vi "Add Entry.vi"(5 "Extra Info":T1, 6 "Parent (None)":string[](array[string]), 7 "Name Prefix (none)":string, 8 "error in (no error)":errorcluster, 9 "Columns":string[](array[string]), 10 "Name":string, 11 "Tree Map in":refnum<class "Tree Map.lvclass">) -> (0 "error out":errorcluster, 3 "Tree Map out":refnum<class "Tree Map.lvclass">, 4 "Hierarchy":string[](array[string]))   [LabVIEW 2020, in "Tree Map.lvlib" / "Tree Map.lvclass"]
uses:
  Tree Map.lvclass
  Extra Entry Info.ctl
  Tree Entry.ctl
  Tree Map.lvclass/Tree Map.ctl
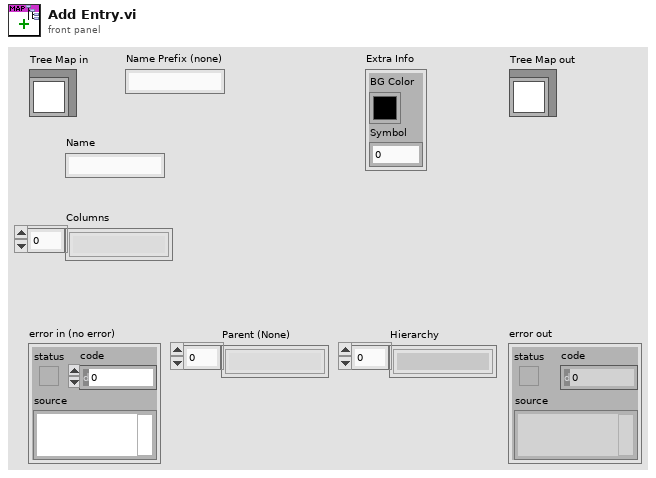
[diagram p1: front panel]
types:
  T1 = typedef "Tree Map.lvlib/Tree Map.lvclass/Extra Entry Info.ctl" = cluster{"BG Color":u32, "Symbol":i32}
  T2 = typedef "Tree Map.lvlib/Tree Map.lvclass/Tree Entry.ctl" = cluster{"Hierarchy":string[], "Name":string, "Columns":string[], "Leaf":bool, "Extra":T1}
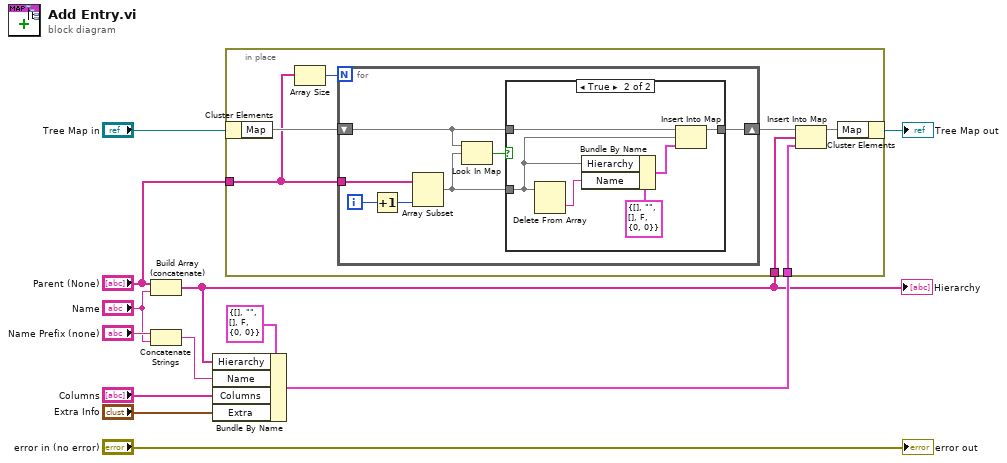
[diagram p0: block diagram]
diagram:
  n1 = Build Array (concatenate)("Parent (None)", "Name") -> (w4:string[])
  "Hierarchy" <- w4
  n2 = Concatenate Strings("Name Prefix (none)", "Name") -> (w8:string)
  n3 = Bundle By Name(cluster=T2 {"Hierarchy"=[], "Name"="", "Columns"=[], "Leaf"=FALSE, "Extra"={"BG Color"=0, "Symbol"=0}} ("Tree Entry"), "Hierarchy"=w4, "Name"=w8, "Columns"="Columns", "Extra"="Extra Info") -> (w5:T2)
  n4 = in-place {
    in-place-border: w5 -> [w19]
    in-place-border: w4 -> [w18]
    in-place-border: "Parent (None)" -> [w14]
    n5 = in-place-cluster #1("Tree Map in") -> ("Map"=w16:map{string[], T2})
    n6 = Array Size(array=w14) -> (size(s)=w13:i32)
    n7 = for {
      N: w13 -> [_]
      shift-right: [w21] -> w15
      shift-left: w16 -> [w23]
      tunnel: w14 -> [w26]
      i -> [w25]
      n8 = Increment(x=w25) -> (x+1=w20:i32)
      n9 = Array Subset(array=w26, length=w20) -> (w22:string[])  [unwired: 1 in]
      n10 = Look In Map(map=w23, key=w22) -> (key not found?=w24:bool)  [unwired: 1 in, 1 out]
      n11 = case shown="True" w24 {
        tunnel: w23 -> [w27 w33]
        tunnel: w22 -> [_ w29]
        tunnel: [w27 w32] -> w21
        frame False {
        }
        frame True {
          n12 = Delete From Array(array=w29) -> (deleted portion=w28:string)  [unwired: 2 in, 1 out]
          n13 = Bundle By Name(cluster=T2 {"Hierarchy"=[], "Name"="", "Columns"=[], "Leaf"=FALSE, "Extra"={"BG Color"=0, "Symbol"=0}} ("value"), "Hierarchy"=w29, "Name"=w28) -> (w30:T2)
          n14 = Insert Into Map(map in=w33, key=w29, value=w30) -> (map out=w32:map{string[], T2})  [unwired: 2 out]
        }
      }
    }
    n15 = Insert Into Map(map in=w15, key=w18, value=w19) -> (map out=w17:map{string[], T2})  [unwired: 2 out]
    n16 = in-place-cluster #1("Map"=w17) -> (→"Tree Map out":refnum<class "Tree Map.lvclass">)
  }
  "error out" <- "error in (no error)"
